vi "Shutdown.vi"(8 "Error In":errorcluster) -> (0 "Error Out":errorcluster)   [LabVIEW 2018, in "Toolkit.lvlib"]
doc: "Writes all remaining log statements to the default log file if enabled and properly closes all files and releases all listeners."
uses:
  Toolkit.lvlib
  Support/File/File Action.ctl
  Support/Error/Error Action.ctl
  Support/Action.ctl
  Support/File/File.lvlib
  Support/Error/Error.lvlib
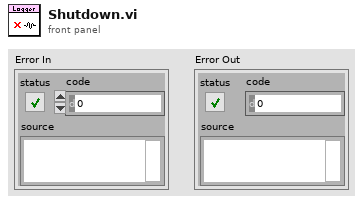
[diagram p1: front panel]
types:
  T1 = typedef "Toolkit.lvlib/File.lvlib/File Action.ctl" = enum16{"Initialize", "Set Maximum File Size", "Set Maximum File Count", "Set Root Folder", "Set Enable Calendar Folder Tree", "Set File Extension", "Start", "Write", "Stop", "Shutdown"}
  T2 = typedef "Toolkit.lvlib/Error.lvlib/Error Action.ctl" = enum16{"Initialize", "Get", "Set Verbosity", "Set User-Defined Codes", "Set User-Defined Descriptions", "Shutdown"}
  T3 = typedef "Toolkit.lvlib/Action.ctl" = enum16{"Initialize", "Register", "Log", "Unregister", "Set Level", "Shutdown"}
  T4 = typedef "Logger.lvlib/Statement.ctl" = cluster{"Time Stamp":timestamp, "Tag":T5, "Source":string, "Message":string}
  T5 = typedef "Logger.lvlib/Tag.ctl" = enum16{"Fatal", "Error", "Warn", "Info", "Debug", "Trace"}
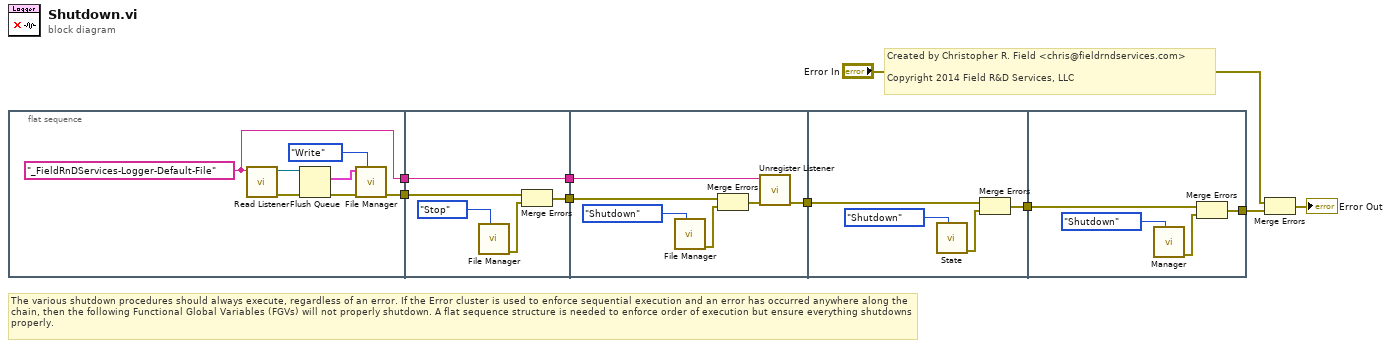
[diagram p0: block diagram]
diagram:
  # "The various shutdown procedures should always execute, regardless of an error. If the Error cluster is used to enforce sequential execution and an error has occurred anywhere along the chain, then the following Functional Global Variables (FGVs) will not properly shutdown. A flat sequence structure is needed to enforce order of execution but ensure everything shutdowns properly."
  # "Created by Christopher R. Field <chris@fieldrndservices.com>\n\nCopyright 2014 Field R&D Services, LLC"
  n1 = flat-sequence {
    tunnel: [w11] -> w5
    tunnel: [w10] -> w3
    tunnel: w5 -> [w19]
    tunnel: [w18] -> w4
    tunnel: w3 -> [w17]
    tunnel: [w17] -> w2
    tunnel: w4 -> [w26]
    tunnel: w2 -> [w23]
    tunnel: [w22] -> w1
    tunnel: [w29] -> w9
    tunnel: w1 -> [w28]
    tunnel: w9 -> [w34]
    tunnel: [w32] -> w8
    frame #0 {
      w10 = "_FieldRnDServices-Logger-Default-File" ("Listener ID")
      n2 = call "Read Listener.vi"("Listener ID"=w10) -> ("Error Out"=w15:errorcluster, "Listener"=w16:refnum<queue>)  [unwired: 9 in]
      n3 = Flush Queue(queue=w16, error in (no error)=w15) -> (remaining elements=w13:T4[], error out=w12:errorcluster)  [unwired: 1 out]
      n4 = call "File Manager.vi"("Action"=File_Action."Write", "Error In"=w12, "Set Value"=w13) -> ("Error Out"=w11:errorcluster)  [unwired: 8 in]
    }
    frame #1 {
      n5 = call "File Manager.vi"("Action"=File_Action."Stop") -> ("Error Out"=w20:errorcluster)  [unwired: 10 in]
      n6 = Merge Errors(w19, w20) -> (w18:errorcluster)
    }
    frame #2 {
      n7 = call "File Manager.vi"("Action"=File_Action."Shutdown") -> ("Error Out"=w25:errorcluster)  [unwired: 10 in]
      n8 = Merge Errors(w26, w25) -> (w24:errorcluster)
      n9 = call "Unregister Listener.vi"("Error In"=w24, "Listener ID"=w23) -> ("Error Out"=w22:errorcluster)  [unwired: 9 in]
    }
    frame #3 {
      n10 = call "State.vi"("Action"=Error_Action."Shutdown") -> ("Error Out"=w30:errorcluster)  [unwired: 9 in, 1 out]
      n11 = Merge Errors(w28, w30) -> (w29:errorcluster)
    }
    frame #4 {
      n12 = call "Manager.vi"("Action"=Action."Shutdown") -> ("Error Out"=w33:errorcluster)  [unwired: 10 in]
      n13 = Merge Errors(w34, w33) -> (w32:errorcluster)
    }
  }
  n14 = Merge Errors("Error In", w8) -> (→"Error Out":errorcluster)
